vi "Generate Compiled Settings Cluster.vi"(7 "Compiled Settings Path":path, 8 "error in":errorcluster, 11 "XML Path":path) -> (0 "error out":errorcluster)   [LabVIEW 2026, in "XML Parser.lvlib"]
uses:
  XML Parser.lvlib
  <resource>/objmgr/DOMUserDefRef.rc
  <vilib>/xml/NI_XML.lvlib
  <vilib>/xml/Close Reference(Node).vi
  <vilib>/xml/Load XML File.vi
panel:
  out "Schema validation errors":string
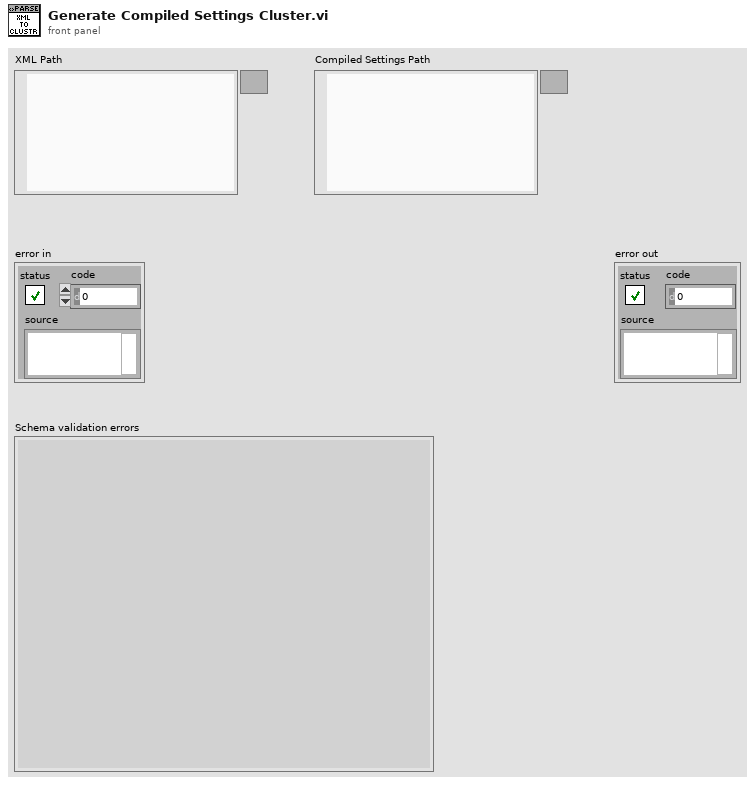
[diagram p1: front panel]
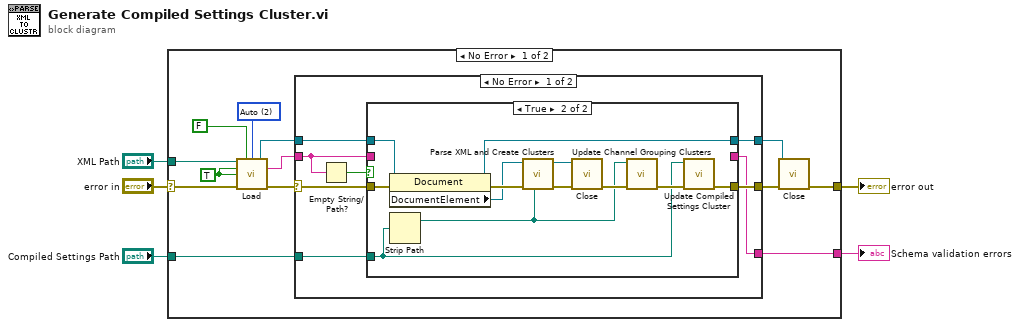
[diagram p0: block diagram]
diagram:
  n1 = case shown="No Error" "error in" {
    selector: "error in" -> [w6 w45]
    tunnel: [w18 w45] -> w5
    tunnel: [w9 _] -> w4
    tunnel: "XML Path" -> [w8 _]
    tunnel: "Compiled Settings Path" -> [w7 _]
    frame No Error {
      w13 = 2 items=["Never", "Always", "Auto"] ("Validate On Load")
      w14 = TRUE ("Do Namespaces")
      n2 = call-poly <vilib>:"Load.vi"("path to XML document"=w8, "preserve whitespace (True)"=FALSE, "validate on load (Auto)"=w13, "process namespaces (False)"=w14, "process schema (False)"=w14, "error in (no error)"=w6) -> ("DOM document out"=w12:refnum<k20>, "parse errors"=w11:string, "error out"=w16:errorcluster)  [unwired: 1 in, 6 out]
      n3 = case shown="No Error" w16 {
        selector: w16 -> [w25 w44]
        tunnel: [w26 w44] -> w17
        tunnel: [w24 w43] -> w15
        tunnel: w12 -> [w23 w43]
        tunnel: w11 -> [w22 w42]
        tunnel: [w19 w42] -> w9
        tunnel: w7 -> [w20 _]
        frame No Error {
          n4 = Empty String/Path?(string/path=w22) -> (empty?=w21:bool)
          n5 = case shown="True" w21 {
            tunnel: w25 -> [w29 w41]
            tunnel: w23 -> [w28 w35]
            tunnel: [w28 w34] -> w24
            tunnel: [w29 w36] -> w26
            tunnel: w22 -> [w27 _]
            tunnel: w20 -> [_ w30]
            tunnel: [w27 _] -> w19
            frame False {
            }
            frame True {
              n6 = property on="Property Node" class="Document"(reference=w35, error in=w41) -> (reference out=w34:refnum<k20>, error out=w40:errorcluster, "DocumentElement"=w33:refnum<k20>)
              n7 = Strip Path(path=w30) -> (stripped path=w31:path)  [unwired: 1 out]
              n8 = call "Parse XML and Create Clusters.vi"("Settings Cluster Path"=w31, "error in"=w40, "Document Element"=w33) -> ("error out"=w39:errorcluster, "Document Element"=w32:refnum<k20>)  [unwired: 7 in]
              n9 = call-poly <vilib>:"Close.vi"("error in (no error)"=w39, "node"=w32) -> ("error out"=w38:errorcluster)  [unwired: 7 in]
              n10 = call "Update Channel Grouping Clusters.vi"("error in"=w38, "Settings Cluster Path"=w31) -> ("error out"=w37:errorcluster)  [unwired: 9 in]
              n11 = call "Update Compiled Settings Cluster.vi"("error in"=w37, "Compiled Settings Path"=w30) -> ("error out"=w36:errorcluster)  [unwired: 9 in]
            }
          }
        }
        frame Error {
        }
      }
      n12 = call-poly <vilib>:"Close.vi"("error in (no error)"=w17, "node"=w15) -> ("error out"=w18:errorcluster)  [unwired: 7 in]
    }
    frame Error {
    }
  }
  "error out" <- w5
  "Schema validation errors" <- w4
